vi "Drive For Distance.vi"(6 "Synchronization":enum16{"Start", "Wait"}(ring), 7 "Description":string, 8 "Command Info In":T1, 9 "Distance":dbl, 10 "Speed":dbl, 11 "Vision":bool) -> (0 "Command Info Out":T1, 3 "Outcome":string="foo")   [LabVIEW 2016]
doc: "This VI sets the motors to run for a given number of seconds. It optionally synchronizes with the completion of the command."
uses:
  <vilib>/Rock Robotics/WPI/Framework/Command Status Info.ctl
  <vilib>/Rock Robotics/WPI/Framework/Completion Status.ctl
  <vilib>/Rock Robotics/WPI/Framework/Completion Notifier.ctl
  Implementation/Drive Setpoints.ctl
  Implementation/Drive Operations.ctl
  Shared/AutoPositions Type Def.ctl
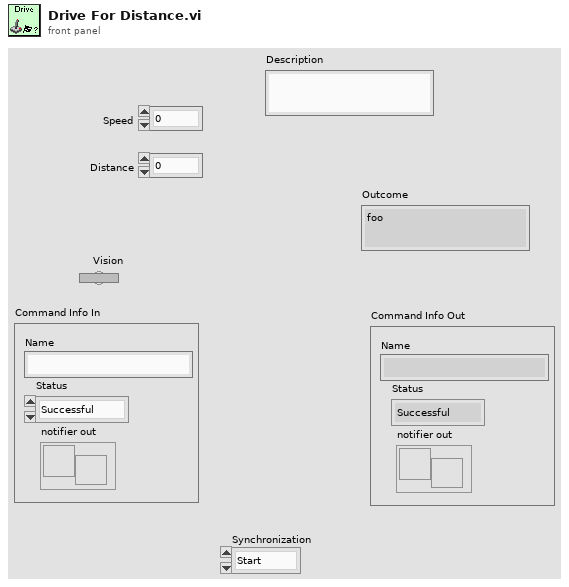
[diagram p1: front panel]
types:
  T1 = typedef "Command Status Info.ctl" = cluster{"Name":string, "Status":T2, "notifier out":T3}
  T2 = typedef "Completion Status.ctl" = enum16{"Successful", "Aborted", "Incomplete"}
  T3 = typedef "Completion Notifier.ctl" = refnum<notifier>
  T4 = typedef "Drive Setpoints.ctl" = cluster{"Operation":T5, "Left Setpoint":dbl, "Right Setpoint":dbl, "Duration":dbl, "Start Position":T6}
  T5 = typedef "Drive Operations.ctl" = enum16{"Reserve", "Read Current", "Immediate", "Drive for Time", "Drive for Distance", "Drive for Angle", "Drive with Angle", "Auto Align", "Auto"}
  T6 = typedef "AutoPositions Type Def.ctl" = enum16{"Left", "Middle", "Right"}
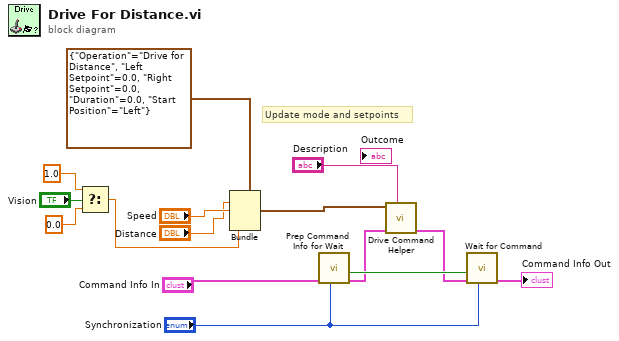
[diagram p0: block diagram]
diagram:
  # "Update mode and setpoints"
  n1 = Select(t=1.0, s="Vision", f=0.0 ("t")) -> (s? t:f=w2:dbl)
  n2 = Bundle(cluster=T4 {"Operation"=enum."Drive for Distance", "Left Setpoint"=0.0, "Right Setpoint"=0.0, "Duration"=0.0, "Start Position"=enum."Left"} ("SubSystem Data"), "Left Setpoint"="Distance", "Right Setpoint"="Speed", "Duration"=w2) -> (w8:T4)  [unwired: 2 in]
  n3 = call <vilib>:"Prep Command Info for Wait.vi"("Synchronication"="Synchronization", "Command Info"="Command Info In") -> ("Command Info"=w12:T1, "Allocated"=w13:bool)  [unwired: 8 in]
  n4 = call "Drive Command Helper.vi"("Description"="Description", "Command Info In"=w12, "SubSystem Data"=w8) -> ("Command Info Out"=w9:T1)  [unwired: 7 in, 1 out]
  n5 = call <vilib>:"Wait for Command.vi"("Synchronication"="Synchronization", "Command Info in"=w9, "Allocated"=w13) -> ("Command Info out"=→"Command Info Out":T1)  [unwired: 8 in]
